vi "Remove_unprintable_Char.vi"(1 "Input String":string="\u0000Hello Fred Bloggs\n\n\u0000") -> (0 "Output String":string)   [LabVIEW 2018]
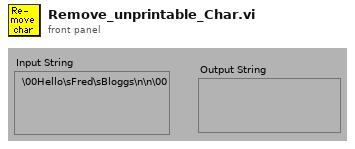
[diagram p1: front panel]
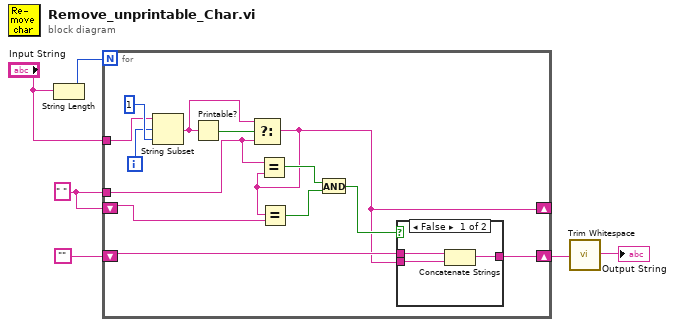
[diagram p0: block diagram]
diagram:
  w3 = " "
  n1 = String Length(string="Input String") -> (length=w6:i32)
  n2 = for {
    N: w6 -> [_]
    tunnel: "Input String" -> [w17]
    shift-right: [w15] -> w2
    shift-left: "" -> [w16]
    shift-right: [w7] -> _
    shift-left: w3 -> [w12]
    tunnel: w3 -> [w8]
    i -> [w18]
    n3 = String Subset(string=w17, offset (0)=w18, length (rest)=1 ("length")) -> (substring=w13:string)
    n4 = Printable?(1:w13) -> (0:w14:bool)
    n5 = Select(t=w13, s=w14, f=w8) -> (s? t:f=w7:string)
    n6 = Equal?(x=w8, y=w7) -> (x = y?=w11:bool)
    n7 = Equal?(x=w7, y=w12) -> (x = y?=w10:bool)
    n8 = And(x=w11, y=w10) -> (x .and. y?=w9:bool)
    n9 = case shown="False" w9 {
      tunnel: w16 -> [w22 w23]
      tunnel: [w21 w23] -> w15
      tunnel: w7 -> [w20 _]
      frame False {
        n10 = Concatenate Strings(w22, w20) -> (w21:string)
      }
      frame True {
      }
    }
  }
  n11 = call <vilib>:"Trim Whitespace.vi"("string"=w2) -> ("trimmed string"=→"Output String":string)  [unwired: 1 in]
